vi "CONEX-LDS Get Low Pass Filter Freq v2.vi"(11 "Connection Cluster in":T1) -> (1 "Frequency":dbl, 3 "Connection Cluster out":T1, 4 "Response":string)   [LabVIEW 2010]
doc: "FD? - Get low pass filter cut off frequency for Kd"
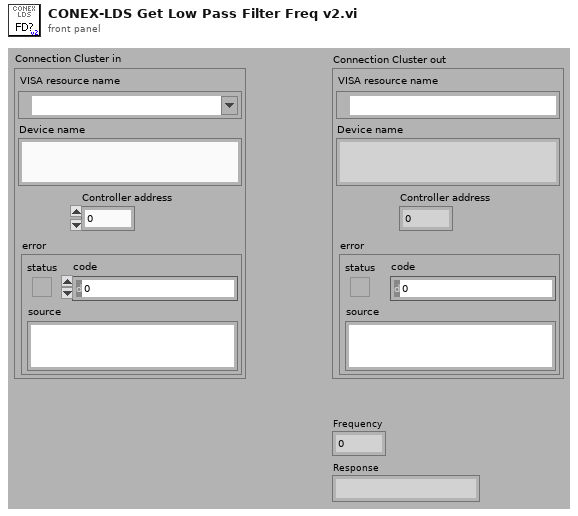
[diagram p1: front panel]
types:
  T1 = cluster{"VISA resource name":refnum<visa-resource-name>, "Device name":string, "Controller address":i32, "error":errorcluster}
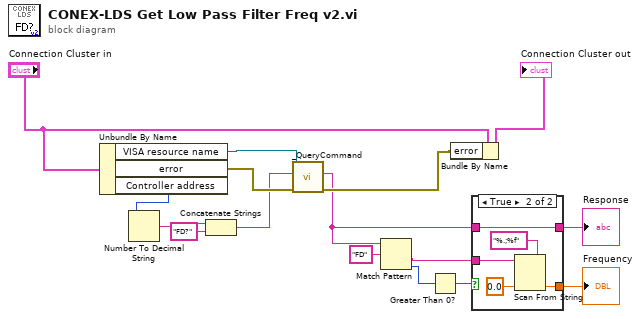
[diagram p0: block diagram]
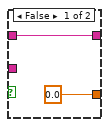
[diagram p2: hidden frame]
diagram:
  n1 = Unbundle By Name("Connection Cluster in") -> ("VISA resource name"=w8:refnum<visa-resource-name>, "error"=w6:errorcluster, "Controller address"=w3:i32)
  n2 = Number To Decimal String(number=w3) -> (decimal integer string=w16:string)  [unwired: 1 out]
  n3 = Concatenate Strings(w16, "FD?" ("strCommand")) -> (w2:string)
  n4 = call <userlib>:"_QueryCommand.vi"("error in"=w6, "Command"=w2, "Instrument Channel in"=w8) -> ("error out"=w7:errorcluster, "Response"=w1:string)  [unwired: 6 in, 1 out]
  n5 = Match Pattern(string=w1, regular expression="FD" ("expression régulière")) -> (after substring=w11:string, offset past match=w12:i32)  [unwired: 3 out]
  n6 = Greater Than 0?(x=w12) -> (x > 0?=w13:bool)
  n7 = Bundle By Name(cluster="Connection Cluster in", "error"=w7) -> (→"Connection Cluster out":T1)
  n8 = case shown="True" w13 {
    tunnel: w1 -> [w18 w20]
    tunnel: w11 -> [_ w21]
    tunnel: [w18 w20] -> w14
    tunnel: [0.0 ("valeur par défaut 1") w19] -> w15
    frame False {
    }
    frame True {
      n9 = Scan From String(format string="%.;%f", input string=w21, default 1=0.0 ("valeur par défaut 1")) -> (output 1=w19:dbl)  [unwired: 2 in, 3 out]
    }
  }
  "Response" <- w14
  "Frequency" <- w15
